vi "Set ExposureTime_us.vi"(8 "error in (no error)":errorcluster, 10 "ExposureTime_us":u32, 11 "TLCamera reference in":refnum<k24>) -> (0 "error out":errorcluster, 3 "TLCamera reference out":refnum<k24>)   [LabVIEW 2015]
uses:
  C:/code/Host/Installer/Scientific Camera Interfaces/LabVIEW/32_bit/Library_X86/Thorlabs.TSI.TLCameraInterfaces.dll
  32_bit/Library_X86/Thorlabs.TSI.TLCameraInterfaces.dll
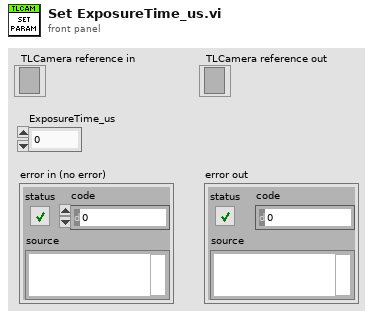
[diagram p1: front panel]
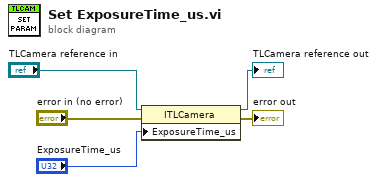
[diagram p0: block diagram]
diagram:
  n1 = property class="ITLCamera"(reference="TLCamera reference in", error in="error in (no error)", "ExposureTime_us"="ExposureTime_us") -> (reference out=→"TLCamera reference out":refnum<k24>, error out=→"error out":errorcluster)
